vi "Ensure Cell is Off.vi"(8 "error in (no error)":errorcluster, 9 "Difficulty":u32, 10 "Category":string, 11 "Grid Screen in":refnum<class "Grid Screen.lvclass">) -> (0 "error out":errorcluster, 3 "Grid Screen out":refnum<class "Grid Screen.lvclass">)   [LabVIEW 2024, in "Grid Screen.lvlib" / "Grid Screen.lvclass"]
uses:
  Grid Screen.lvclass
  Grid Screen.lvclass/Grid Screen.ctl
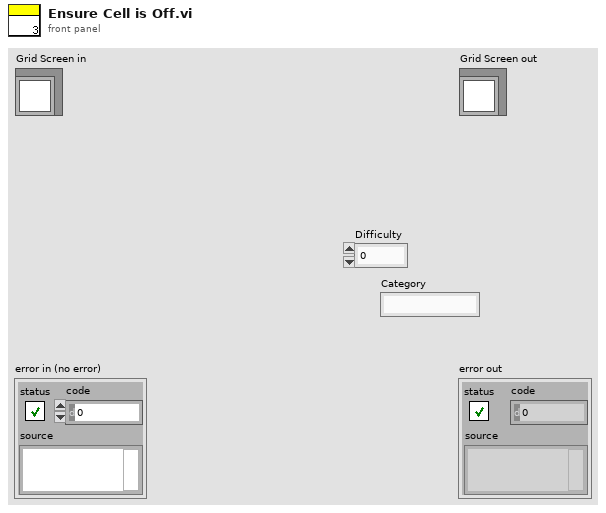
[diagram p1: front panel]
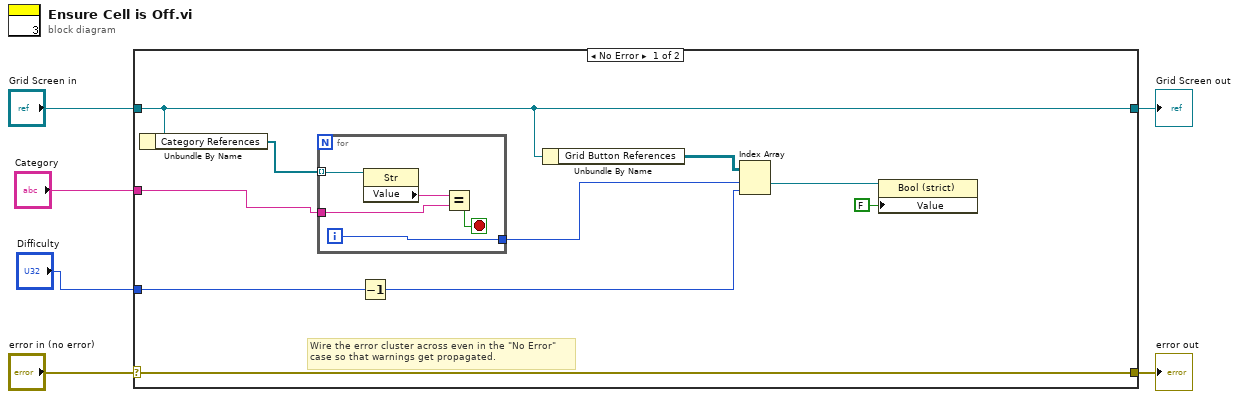
[diagram p0: block diagram]
diagram:
  n1 = case shown="No Error" "error in (no error)" {
    selector: "error in (no error)" -> [w16 w23]
    tunnel: [w16 w23] -> w5
    tunnel: [w13 w22] -> w3
    tunnel: "Grid Screen in" -> [w13 w22]
    tunnel: "Category" -> [w14 _]
    tunnel: "Difficulty" -> [w10 _]
    frame No Error {
      # "Wire the error cluster across even in the \"No Error\"\ncase so that warnings get propagated."
      n2 = Unbundle By Name(w13) -> ("Category References"=w15:refnum<vi>[])
      n3 = for {
        tunnel: w15 -> [w21] mode=indexing
        tunnel: w14 -> [w19]
        tunnel: [w17] -> w11
        i -> [w17]
        stop <- w18 stop-if-true
        n4 = property class="Str"(reference=w21) -> ("Value"=w20:string)  [unwired: 1 in, 2 out]
        n5 = Equal?(x=w20, y=w19) -> (x = y?=w18:bool)
      }
      n6 = Decrement(x=w10) -> (x-1=w9:u32)
      n7 = Unbundle By Name(w13) -> ("Grid Button References"=w12:refnum<vi>[][])
      n8 = Index Array(array=w12, index (row)=w11, index (col)=w9) -> (element=w8:refnum<vi>)
      n9 = property class="Bool (strict)"(reference=w8, "Value"=FALSE) -> ()  [unwired: 1 in, 2 out]
    }
    frame Error {
    }
  }
  "error out" <- w5
  "Grid Screen out" <- w3
